vi "Automation Settings Dialog.vi"(8 "error in (no error)":errorcluster, 11 "Filename":string="data020") -> (0 "error out":errorcluster, 2 "Cancelled?":bool=TRUE, 3 "Settings Out":T1)   [LabVIEW 2013, in "Automation.lvlib"]
uses:
  Automation.lvlib
  Zscan Settings.ctl
panel:
  in  "First data file number:":i32
  in  "Autofill 2 button":bool
  in  "Max Cap Height":dbl=0.1
  in  "Num. Steps":i32=5
  in  "Min Cap Height":dbl=12.0
  in  "Autofill 1 button":bool
  out "Num. Steps":i32=5
  in  "Seconds per Height":i32=100000 format="%^#.2e"
  in  "Delta":dbl=0.1
  in  "Heights":dbl[](array[numeric])
  in  "Num. Steps":i32=5
  in  "Min Cap Height":dbl=12.0
  in  "Cancel Button":bool
  in  "OK Button":bool
  # "MAKE SURE MAX. SAMPLES IS BIG ENOUGH"
  # "Auto Fill 1"
  # "Auto Fill 2"
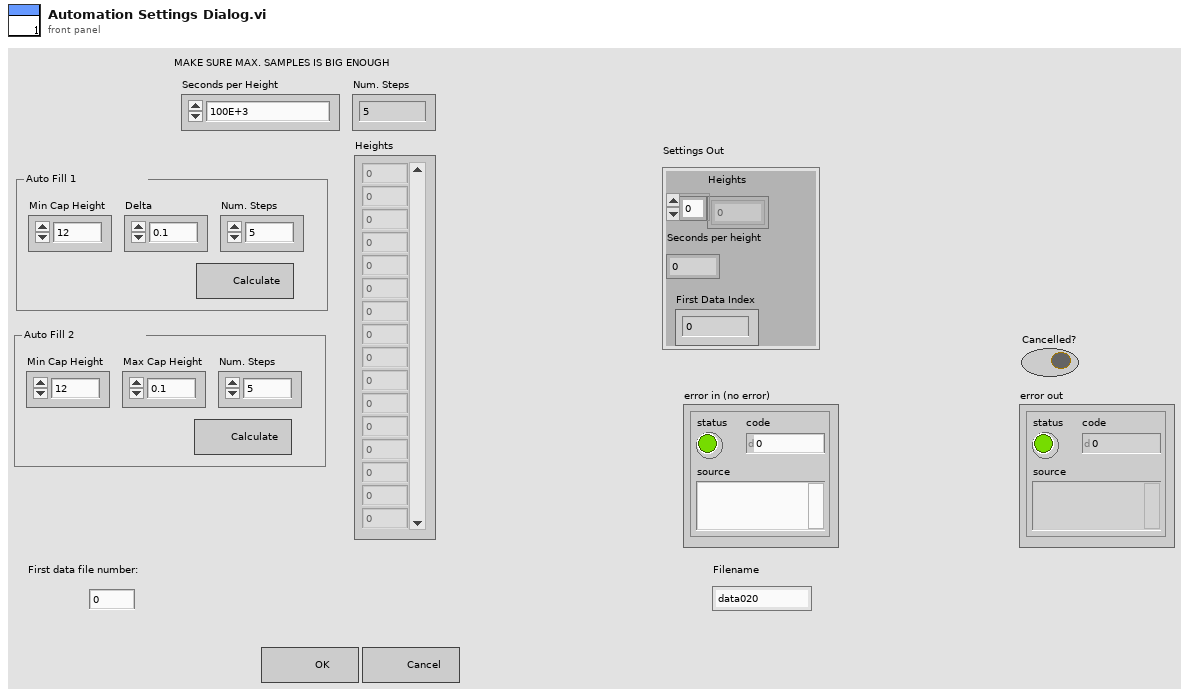
[diagram p1: front panel]
types:
  T1 = typedef "Automation.lvlib/Zscan Settings.ctl" = cluster{"Heights":dbl[], "Seconds per height":i32, "First Data Index":i32}
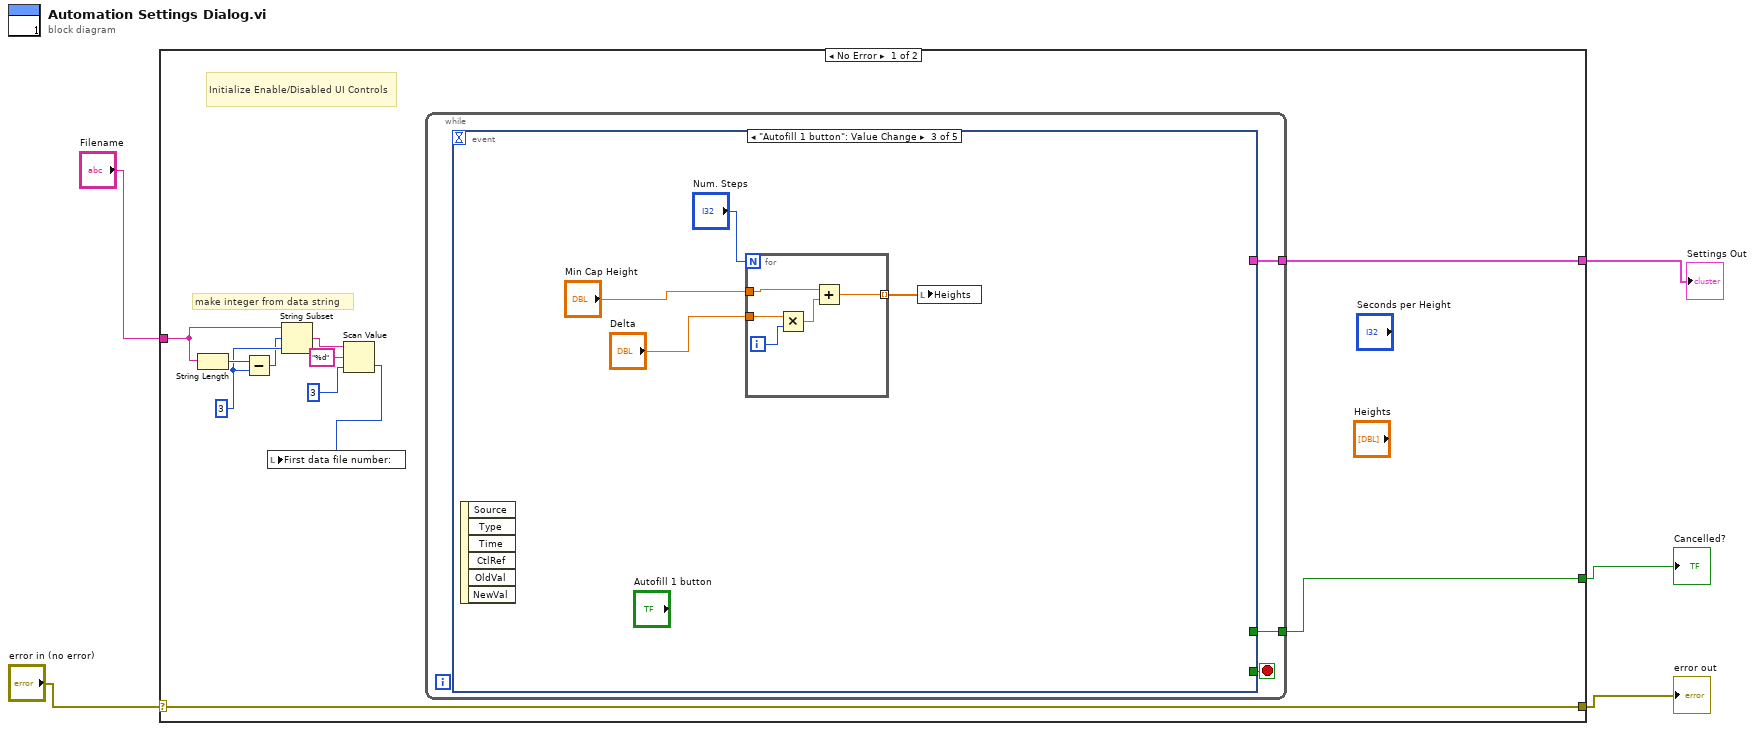
[diagram p0: block diagram]
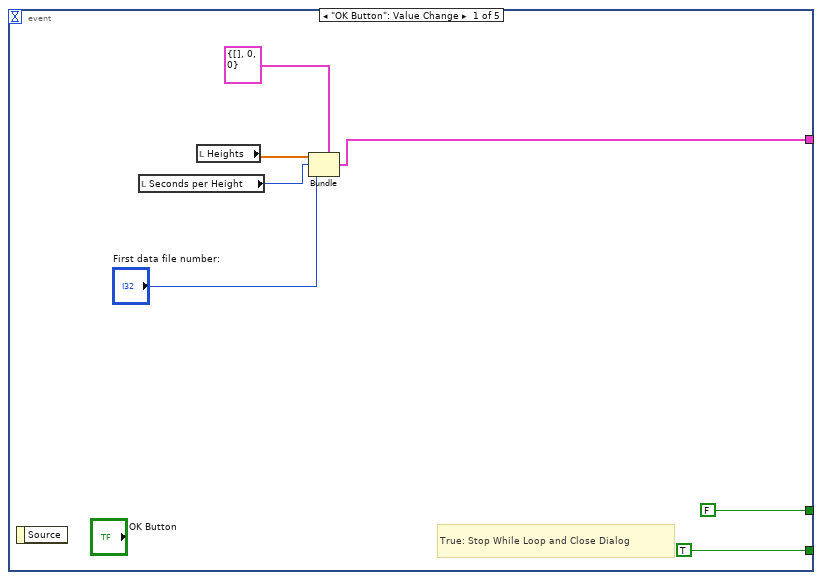
[diagram p2: hidden frame]
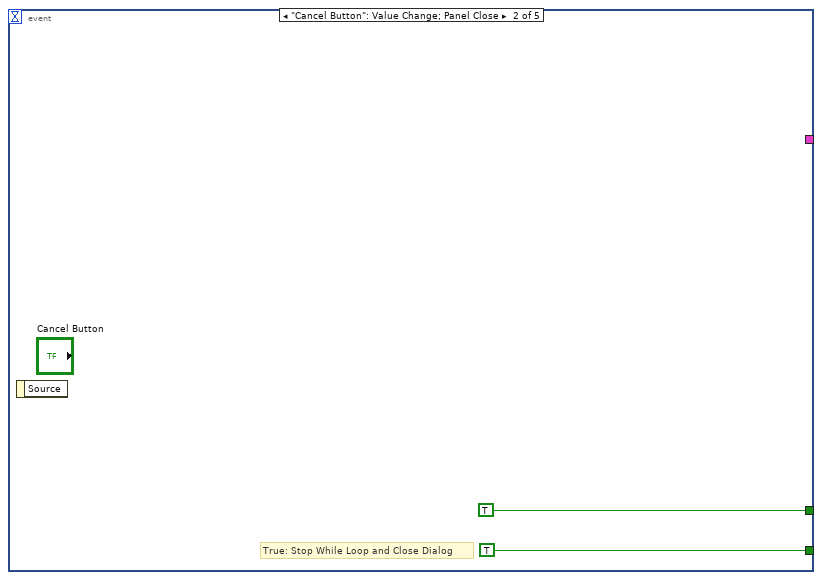
[diagram p3: hidden frame]
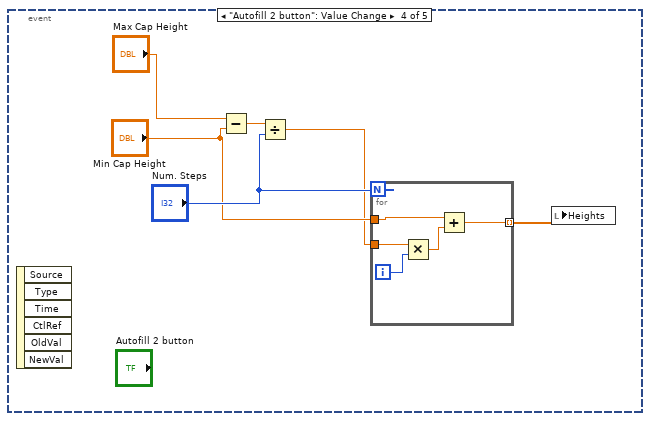
[diagram p4: hidden frame]
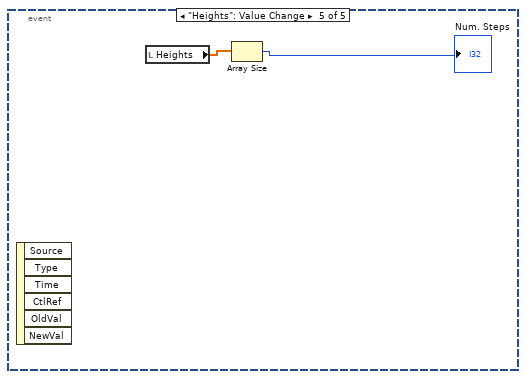
[diagram p5: hidden frame]
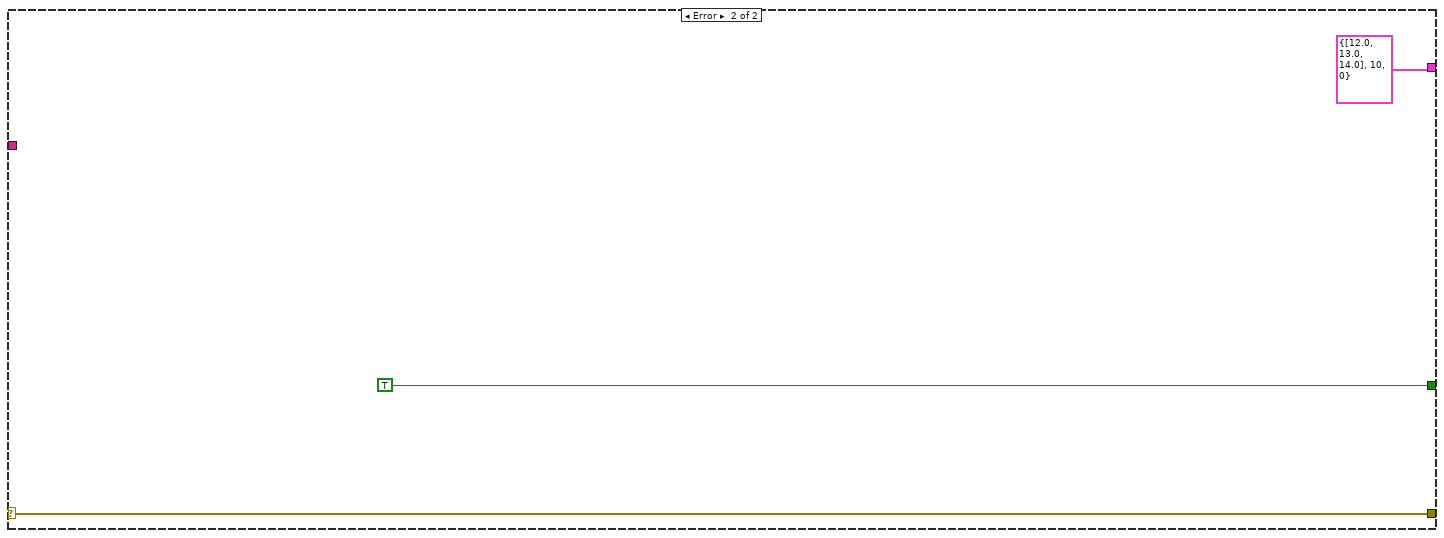
[diagram p6: hidden frame]
diagram:
  n1 = case shown="No Error" "error in (no error)" {
    selector: "error in (no error)" -> [w16 w53]
    tunnel: [w16 w53] -> w4
    tunnel: [w15 TRUE ("UI Refresh Needed?")] -> w5
    tunnel: [w14 T1 {"Heights"=[12.0, 13.0, 14.0], "Seconds per height"=10, "First Data Index"=0} ("Settings Out 2")] -> w2
    tunnel: "Filename" -> [w7 _]
    frame No Error {
      w12 = 3 ("length (rest)")
      # "make integer from data string"
      # "Initialize Enable/Disabled UI Controls"
      n2 = String Length(string=w7) -> (length=w13:i32)
      n3 = Subtract(x=w13, y=w12) -> (x-y=w11:i32)
      n4 = String Subset(string=w7, offset (0)=w11, length (rest)=w12) -> (substring=w10:string)
      n5 = Scan Value(string=w10, format string="%d", default (0 dbl)=3 ("length (rest)")) -> (value=w6:i32)  [unwired: 1 out]
      n6 = local write "First data file number:"(w6) -> ()
      n7 = while {
        tunnel: [w19] -> w15
        tunnel: [w17] -> w14
        stop <- w18 stop-if-true
        n8 = event shown="[2] \"Autofill 1 button\": Value Change" {
          selector: _ -> [_ _ _ _ _]
          dyn-events: _ -> [_ _ _ _ _]
          timeout: _ -> [_ _ _ _ _]
          tunnel: [FALSE ("UI Refresh Needed?") TRUE ("UI Refresh Needed?") _ _ _] -> w19
          tunnel: [TRUE TRUE _ _ _] -> w18
          tunnel: [w22 _ _ _ _] -> w17
          event "OK Button": Value Change {
            # "True: Stop While Loop and Close Dialog"
            n9 = event-data() -> ()  [unwired: 1 in, 1 out]
            n10 = local read "Seconds per Height"() -> (w23:i32)
            n11 = local read "Heights"() -> (w24:dbl[])
            n12 = Bundle(cluster=T1 {"Heights"=[], "Seconds per height"=0, "First Data Index"=0} ("ZScan Settings"), "Heights"=w24, "Seconds per height"=w23, "First Data Index"="First data file number:") -> (w22:T1)
          }
          event "Cancel Button": Value Change; Panel Close {
            # "True: Stop While Loop and Close Dialog"
            n13 = event-data() -> ()  [unwired: 1 in, 1 out]
          }
          event "Autofill 1 button": Value Change {
            n14 = event-data() -> ()  [unwired: 1 in, 6 out]
            n15 = for {
              N: "Num. Steps" -> [_]
              tunnel: "Delta" -> [w37]
              tunnel: "Min Cap Height" -> [w34]
              tunnel: [w33] -> w29 mode=indexing
              i -> [w36]
              n16 = Multiply(x=w37, y=w36) -> (x*y=w35:dbl)
              n17 = Add(x=w34, y=w35) -> (x+y=w33:dbl)
            }
            n18 = local write "Heights"(w29) -> ()
          }
          event "Autofill 2 button": Value Change {
            n19 = event-data() -> ()  [unwired: 1 in, 6 out]
            n20 = Subtract(x="Max Cap Height", y="Min Cap Height") -> (x-y=w42:dbl)
            n21 = Divide(x=w42, y="Num. Steps") -> (x/y=w39:dbl)
            n22 = for {
              N: "Num. Steps" -> [_]
              tunnel: w39 -> [w48]
              tunnel: "Min Cap Height" -> [w45]
              tunnel: [w44] -> w38 mode=indexing
              i -> [w47]
              n23 = Multiply(x=w48, y=w47) -> (x*y=w46:dbl)
              n24 = Add(x=w45, y=w46) -> (x+y=w44:dbl)
            }
            n25 = local write "Heights"(w38) -> ()
          }
          event "Heights": Value Change {
            n26 = event-data() -> ()  [unwired: 1 in, 6 out]
            n27 = local read "Heights"() -> (w50:dbl[])
            n28 = Array Size(array=w50) -> (size(s)=→"Num. Steps":i32)
          }
        }
      }
    }
    frame Error {
    }
  }
  "error out" <- w4
  "Cancelled?" <- w5
  "Settings Out" <- w2
